vi "Launch Server.vi"   [LabVIEW 2020]
uses:
  LV Chat Server/LV Chat Server.lvclass
panel:
  # "1. Run this VI to start the server.\n2. This VI will remain running but hidden while the server is active."
types:
  T1 = enum32{"Invalid", "Standard", "Closed", "Hidden", "Minimized", "Maximized"}
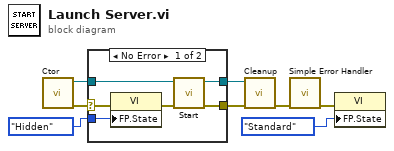
[diagram p0: block diagram]
diagram:
  n1 = call "Ctor.vi"() -> ("error out"=w8:errorcluster, "LV Chat Server out"=w7:refnum<class "LV Chat Server.lvclass">)  [unwired: 10 in]
  n2 = case shown="No Error" w8 {
    selector: w8 -> [w12 w15]
    tunnel: w7 -> [w10 w16]
    tunnel: [w14 w16] -> w6
    tunnel: [w13 w15] -> w5
    tunnel: T1."Hidden" ("Front Panel Window:State") -> [w9 _]
    frame No Error {
      n3 = property class="VI"(error in=w12, "FP.State"=w9) -> (error out=w11:errorcluster)  [unwired: 1 in, 1 out]
      n4 = call "Start.vi"("error in (no error)"=w11, "LV Chat Server in"=w10) -> ("error out"=w13:errorcluster, "LV Chat Server out"=w14:refnum<class "LV Chat Server.lvclass">)  [unwired: 8 in]
    }
    frame Error {
    }
  }
  n5 = call "Cleanup.vi"("error in (no error)"=w5, "LV Chat Server in"=w6) -> ("error out"=w4:errorcluster)  [unwired: 9 in]
  n6 = call <vilib>:"Simple Error Handler.vi"("error in (no error)"=w4) -> ("error out"=w2:errorcluster)  [unwired: 4 in, 4 out]
  n7 = property class="VI"(error in=w2, "FP.State"=T1."Standard" ("Front Panel Window:State")) -> ()  [unwired: 1 in, 2 out]
